vi "Volatus Group Info.vi"(8 "error in (no error)":errorcluster, 11 "Volatus Group":refnum<class "Group.lvclass">) -> (0 "error out":errorcluster, 3 "Group Info":T1)   [LabVIEW 2020, in "Volatus.lvlib"]
uses:
  Volatus.lvlib
  lv-vecto/Vecto/Group Info.ctl
  lv-vecto/Vecto/Vecto.lvlib
  VolatusConfig/Group/Group.lvclass
  VolatusConfig/VolatusConfigElement/VolatusConfigElement.lvclass
  C:/dev/lv20CE/relink/lv-volatus/VolatusConfig/VolatusConfigElement/VolatusConfigElement.lvclass
  C:/dev/lv20CE/relink/lv-volatus/VolatusConfig/Group/Group.lvclass
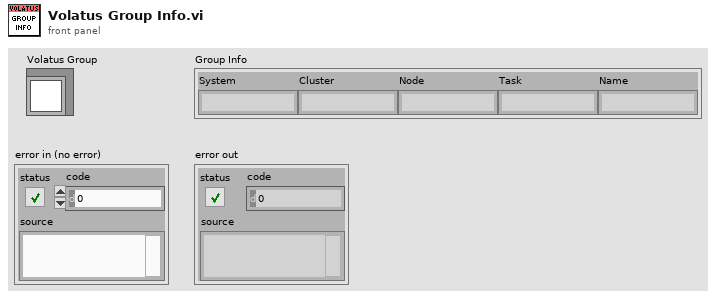
[diagram p1: front panel]
types:
  T1 = typedef "Vecto.lvlib/Group Info.ctl" = cluster{"System":string, "Cluster":string, "Node":string, "Task":string, "Name":string}
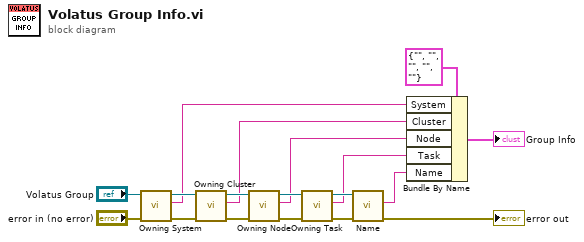
[diagram p0: block diagram]
diagram:
  n1 = call "Owning System.vi"("error in (no error)"="error in (no error)", "Group in"="Volatus Group") -> ("error out"=w4:errorcluster, "Owning System"=w1:string, "Group out"=w2:refnum<class "Group.lvclass">)  [unwired: 7 in]
  n2 = call "Owning Cluster.vi"("error in (no error)"=w4, "Group in"=w2) -> ("error out"=w7:errorcluster, "Owning Cluster"=w5:string, "Group out"=w6:refnum<class "Group.lvclass">)  [unwired: 7 in]
  n3 = call "Owning Node.vi"("error in (no error)"=w7, "Group in"=w6) -> ("error out"=w10:errorcluster, "Owning Node"=w8:string, "Group out"=w9:refnum<class "Group.lvclass">)  [unwired: 7 in]
  n4 = call "Owning Task.vi"("error in (no error)"=w10, "Group in"=w9) -> ("error out"=w13:errorcluster, "Owning Task"=w11:string, "Group out"=w12:refnum<class "Group.lvclass">)  [unwired: 7 in]
  n5 = call "Name.vi"("error in (no error)"=w13, "VolatusConfigElement in"=w12) -> ("error out"=→"error out":errorcluster, "Name"=w14:string)  [unwired: 7 in, 1 out]
  n6 = Bundle By Name(cluster=T1 {"System"="", "Cluster"="", "Node"="", "Task"="", "Name"=""} ("Group Info"), "System"=w1, "Cluster"=w5, "Node"=w8, "Task"=w11, "Name"=w14) -> (→"Group Info":T1)
